vi "DigitalPulse.vi"() -> ()   [LabVIEW 2017]
uses:
  <vilib>/DAQmx/create/channels.llb/DAQmx Create Channel (CO-Pulse Generation-Time).vi
  <vilib>/DAQmx/configure/trigger.llb/DAQmx Start Trigger (Digital Edge).vi
  <resource>/objmgr/daqmx.rc
panel:
  in  "?":T1={"Pulse Width High"=0.001, "counter"="Dev6/ctr0", "Output Terminal"="/Dev6/PFI12", "source"="/Dev6/PFI15", "low time"=0.01} {"low time" min=1e-09 max=5.0 format="%.1e"; "Pulse Width High" min=1e-09 max=5.0}
  in  "stop":bool
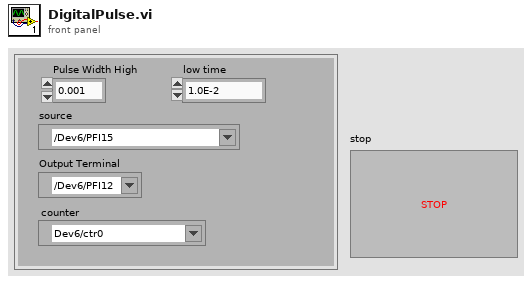
[diagram p1: front panel]
types:
  T1 = cluster{"Pulse Width High":dbl, "counter":tag, "Output Terminal":tag, "source":tag, "low time":dbl}
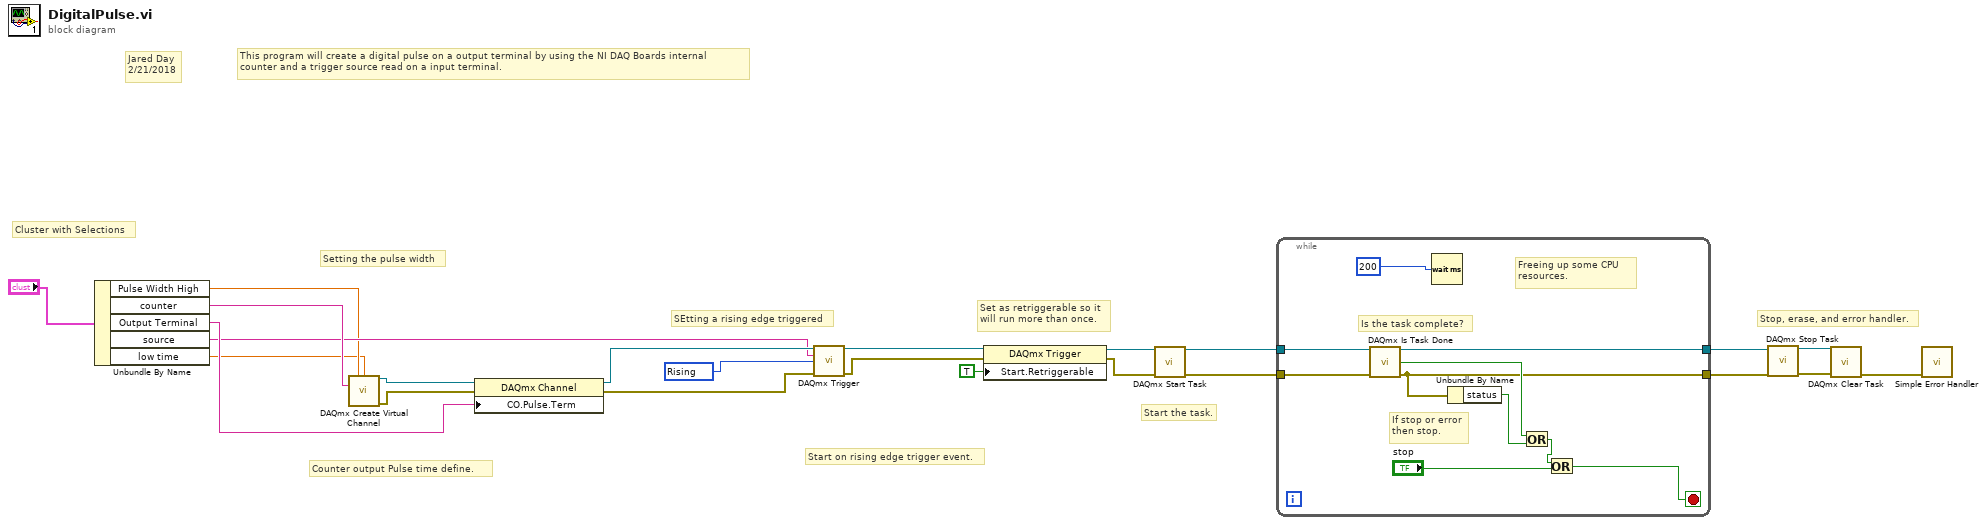
[diagram p0: block diagram]
diagram:
  w16 = 10280 items=["Rising"=10280, "Falling"=10171] ("edge")
  # "Stop, erase, and error handler."
  # "Start the task."
  # "Set as retriggerable so it \nwill run more than once."
  # "Start on rising edge trigger event."
  # "SEtting a rising edge triggered"
  # "Counter output Pulse time define."
  # "Setting the pulse width"
  # "Cluster with Selections"
  # "This program will create a digital pulse on a output terminal by using the NI DAQ Boards internal\ncounter and a trigger source read on a input terminal."
  # "Jared Day\n2/21/2018"
  n1 = Unbundle By Name("?") -> ("Pulse Width High"=w3:dbl, "counter"=w22:tag, "Output Terminal"=w20:tag, "source"=w17:tag, "low time"=w1:dbl)
  n2 = call-poly <vilib>:"DAQmx Create Virtual Channel.vi"("high time"=w3, "low time"=w1, "counter"=w22) -> ("task out"=w21:refnum<k21>, "error out"=w19:errorcluster)  [unwired: 11 in]
  n3 = property class="DAQmx Channel"(reference=w21, error in=w19, "CO.Pulse.Term"=w20) -> (reference out=w18:refnum<k21>, error out=w2:errorcluster)
  n4 = call-poly <vilib>:"DAQmx Trigger.vi"("task/channels in"=w18, "source"=w17, "edge"=w16, "error in"=w2) -> ("task out"=w15:refnum<k21>, "error out"=w14:errorcluster)  [unwired: 10 in]
  n5 = property class="DAQmx Trigger"(reference=w15, error in=w14, "Start.Retriggerable"=TRUE) -> (reference out=w12:refnum<k21>, error out=w11:errorcluster)
  n6 = call <vilib>:"DAQmx Start Task.vi"("task/channels in"=w12, "error in"=w11) -> ("task out"=w10:refnum<k21>, "error out"=w9:errorcluster)  [unwired: 12 in]
  n7 = while {
    tunnel: w10 -> [w32]
    tunnel: w9 -> [w31]
    tunnel: [w25] -> w7
    tunnel: [w24] -> w8
    stop <- w28 stop-if-true
    # "Is the task complete?"
    # "If stop or error\nthen stop."
    # "Freeing up some CPU \nresources."
    n8 = call <vilib>:"DAQmx Is Task Done.vi"("task/channels in"=w32, "error in"=w31) -> ("task out"=w24:refnum<k21>, "task done?"=w26:bool, "error out"=w25:errorcluster)  [unwired: 11 in]
    n9 = Wait (ms)(milliseconds to wait=200) -> ()  [unwired: 1 out]
    n10 = Unbundle By Name(w25) -> ("status"=w27:bool)
    n11 = Or(x=w26, y=w27) -> (x .or. y?=w29:bool)
    n12 = Or(x=w29, y="stop") -> (x .or. y?=w28:bool)
  }
  n13 = call <vilib>:"DAQmx Stop Task.vi"("task/channels in"=w8, "error in"=w7) -> ("task out"=w6:refnum<k21>, "error out"=w5:errorcluster)  [unwired: 12 in]
  n14 = call <vilib>:"DAQmx Clear Task.vi"("task in"=w6, "error in"=w5) -> ("error out"=w4:errorcluster)  [unwired: 13 in]
  n15 = call <vilib>:"Simple Error Handler.vi"("error in (no error)"=w4) -> ()  [unwired: 4 in, 5 out]
